vi "Wait.vi"(8 "error in (no error)":errorcluster, 11 "Timer in":refnum<class "Timer.lvclass">) -> (0 "error out":errorcluster, 1 "elapsed time(s)":dbl, 2 "timeout":bool, 3 "Timer out":refnum<class "Timer.lvclass">)   [LabVIEW 2020, in "Timer.lvclass"]
uses:
  Timer.lvclass
  Timer.lvclass/Timer.ctl
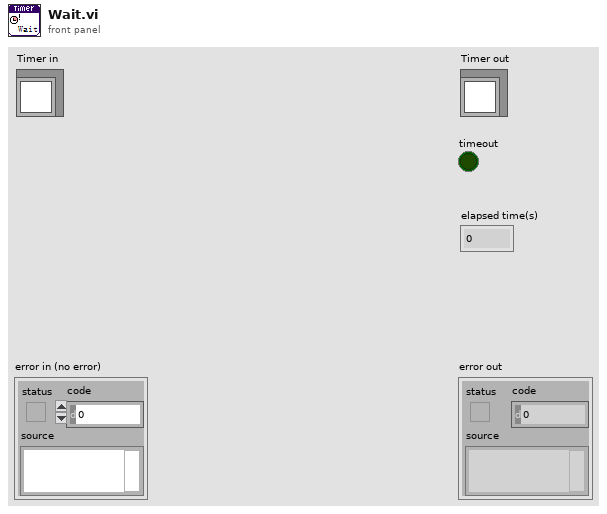
[diagram p1: front panel]
types:
  T1 = cluster{"target time(ms)":u32, "elapsed time(ms)":u32, "start time":u32, "pause":bool}
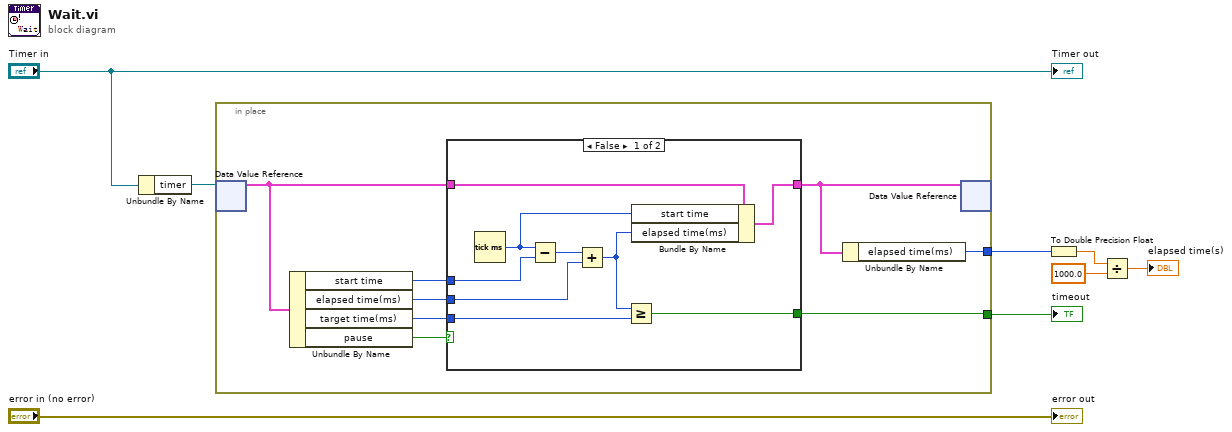
[diagram p0: block diagram]
diagram:
  n1 = Unbundle By Name("Timer in") -> ("timer"=w1:refnum<data-value>)
  n2 = in-place {
    in-place-border: [w11] -> w6
    in-place-border: [w9] -> w5
    n3 = in-place-dvr #1(w1) -> (w16:T1)  [unwired: 1 out]
    n4 = Unbundle By Name(w16) -> ("start time"=w12:u32, "elapsed time(ms)"=w13:u32, "target time(ms)"=w14:u32, "pause"=w15:bool)
    n5 = case shown="False" w15 {
      tunnel: w12 -> [w25 _]
      tunnel: w13 -> [w18 _]
      tunnel: [w24 _] -> w11
      tunnel: w14 -> [w17 _]
      tunnel: w16 -> [w23 w26]
      tunnel: [w20 w26] -> w10
      frame False {
        n6 = Tick Count (ms)() -> (millisecond timer value=w21:u32)
        n7 = Subtract(x=w21, y=w25) -> (x-y=w19:u32)
        n8 = Add(x=w19, y=w18) -> (x+y=w22:u32)
        n9 = Greater Or Equal?(x=w22, y=w17) -> (x >= y?=w24:bool)
        n10 = Bundle By Name(cluster=w23, "start time"=w21, "elapsed time(ms)"=w22) -> (w20:T1)
      }
      frame True {
      }
    }
    n11 = Unbundle By Name(w10) -> ("elapsed time(ms)"=w9:u32)
    n12 = in-place-dvr #1(w10) -> ()  [unwired: 2 out]
  }
  "timeout" <- w6
  n13 = To Double Precision Float(number=w5) -> (double precision float=w4:dbl)
  n14 = Divide(x=w4, y=1000.0) -> (x/y=→"elapsed time(s)":dbl)
  "error out" <- "error in (no error)"
  "Timer out" <- "Timer in"
